vi "Read Groups.vi"(8 "error in (no error)":errorcluster, 11 "Blackboard in":refnum<class "Blackboard.lvclass">) -> (0 "error out":errorcluster, 2 "Groups":refnum<data-value>, 3 "Blackboard out":refnum<class "Blackboard.lvclass">)   [LabVIEW 2021, in "Blackboard.lvclass"]
uses:
  Blackboard.lvclass
  Blackboard.lvclass/Blackboard.ctl
  Support/Tags Map Type.ctl
  Support/Data Type.ctl
  Support/Status Type.ctl
  Support/Data DVR Type.ctl
  Support/Group Map Type.ctl
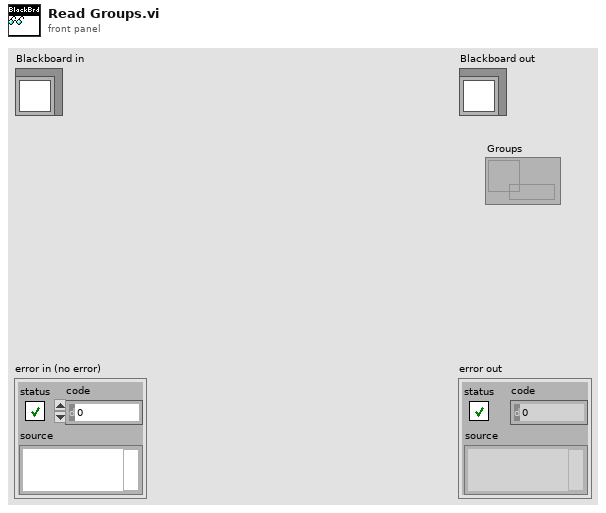
[diagram p1: front panel]
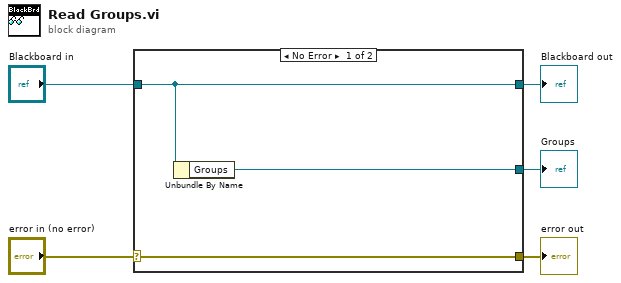
[diagram p0: block diagram]
diagram:
  n1 = case shown="No Error" "error in (no error)" {
    selector: "error in (no error)" -> [w8 w9]
    tunnel: [w8 w9] -> w4
    tunnel: [w7 w10] -> w2
    tunnel: "Blackboard in" -> [w7 w10]
    tunnel: [w6 _] -> w1
    frame No Error {
      n2 = Unbundle By Name(w7) -> ("Groups"=w6:refnum<data-value>)
    }
    frame Error {
    }
  }
  "error out" <- w4
  "Blackboard out" <- w2
  "Groups" <- w1
